vi "Get_VI_margin_settings.vi"(0 "reference":refnum<vi>, 1 "error in (no error)":errorcluster) -> (2 "reference out":refnum<vi>, 3 "Margin":T1={"override VI margins (false)"=FALSE, "margins (1.00)"={"top"=1.0, "left"=1.0, "right"=1.0, "bottom"=1.0}, "measurement system (default)"=0} {"measurement system (default)" items=["Default", "US", "Metric"]; "margins (1.00)"."right" format="%.2f"; "margins (1.00)"."bottom" format="%.2f"; "margins (1.00)"."top" format="%.2f"; "margins (1.00)"."left" format="%.2f"}, 4 "error out":errorcluster)   [LabVIEW 2017, in "NI_ReportGenerationCore.lvlib"]
uses:
  <vilib>/Utility/NIReport.llb/NI_ReportGenerationCore.lvlib
  <vilib>/printing/EasyPrintingControls.llb/margins.ctl
  <vilib>/printing/EasyPrintingControls.llb/margin_values.ctl
  <vilib>/printing/EasyPrintingControls.llb/measurement_system.ctl
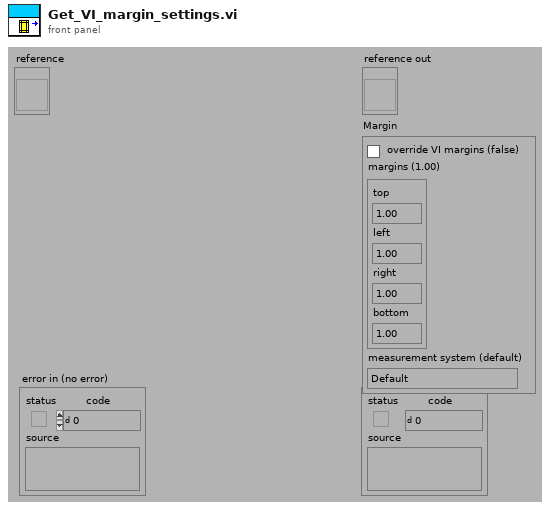
[diagram p1: front panel]
types:
  T1 = typedef "NI_ReportGenerationCore.lvlib/margins.ctl" = cluster{"override VI margins (false)":bool, "margins (1.00)":T2, "measurement system (default)":T3}
  T2 = typedef "NI_ReportGenerationCore.lvlib/margin_values.ctl" = cluster{"top":dbl, "left":dbl, "right":dbl, "bottom":dbl}
  T3 = typedef "NI_ReportGenerationCore.lvlib/measurement_system.ctl" = u16
  T4 = typedef "LVPrintingMarginsTypeDef.ctl" = cluster{"Top":sgl, "Left":sgl, "Bottom":sgl, "Right":sgl, "Measurement System":enum8{"Inches", "cm"}}
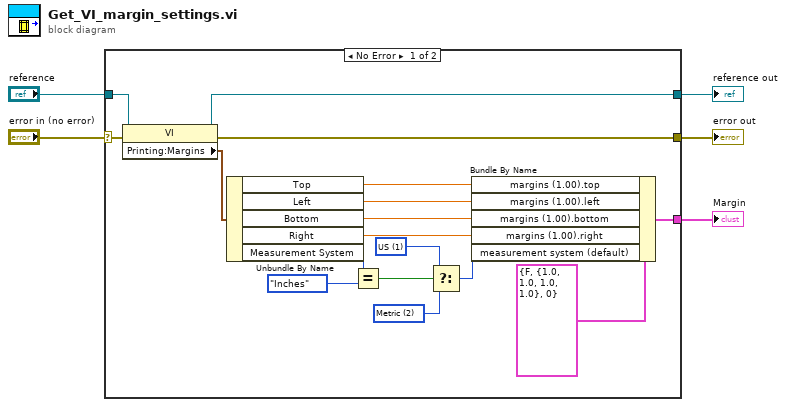
[diagram p0: block diagram]
diagram:
  n1 = case shown="No Error" "error in (no error)" {
    selector: "error in (no error)" -> [w21 w23]
    tunnel: "reference" -> [w7 w24]
    tunnel: [w6 w24] -> w2
    tunnel: [w22 w23] -> w5
    tunnel: [w8 _] -> w1
    frame No Error {
      w9 = T3 2 items=["Default", "US", "Metric"] ("measurement system (default)")
      w10 = T3 1 items=["Default", "US", "Metric"] ("measurement system (default)")
      n2 = property class="VI"(reference=w7, error in=w21) -> (reference out=w6:refnum<vi>, error out=w22:errorcluster, "Printing:Margins"=w16:T4)
      n3 = Unbundle By Name(w16) -> ("Top"=w20:sgl, "Left"=w19:sgl, "Bottom"=w18:sgl, "Right"=w17:sgl, "Measurement System"=w14:enum8{"Inches", "cm"})
      n4 = Equal?(x=w14, y=enum8{"Inches", "cm"}."Inches" ("measurement system")) -> (x = y?=w13:bool)
      n5 = Select(t=w10, s=w13, f=w9) -> (s? t:f=w12:T3)
      n6 = Bundle By Name(cluster=T1 {"override VI margins (false)"=FALSE, "margins (1.00)"={"top"=1.0, "left"=1.0, "right"=1.0, "bottom"=1.0}, "measurement system (default)"=0} ("margins"), "margins (1.00).top"=w20, "margins (1.00).left"=w19, "margins (1.00).bottom"=w18, "margins (1.00).right"=w17, "measurement system (default)"=w12) -> (w8:T1)
    }
    frame Error {
    }
  }
  "error out" <- w5
  "reference out" <- w2
  "Margin" <- w1
